vi "Exercise1_Week2.vi"() -> ()   [LabVIEW 2015]
panel:
  out "Output Fibonacci":dbl
  in  "Input Fibonacci":dbl
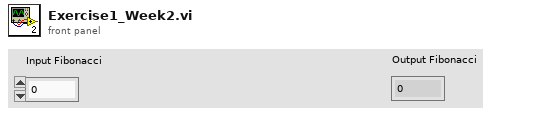
[diagram p1: front panel]
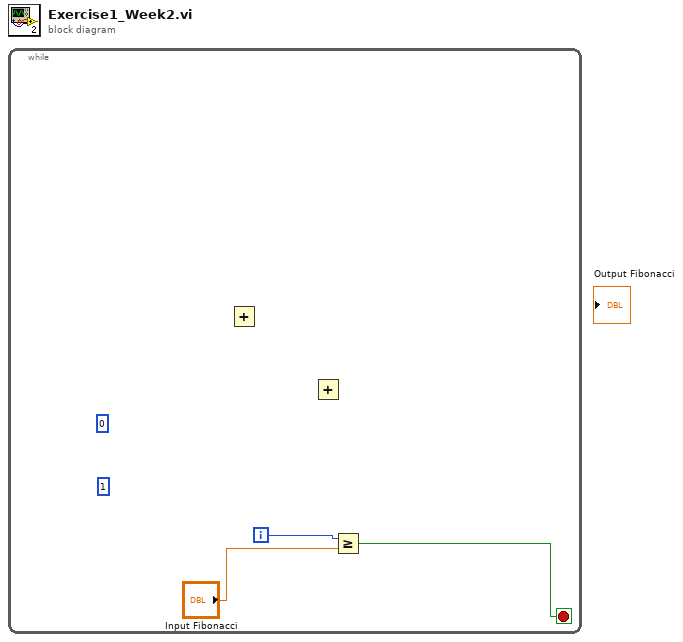
[diagram p0: block diagram]
diagram:
  n1 = while {
    i -> [w2]
    stop <- w3 stop-if-true
    (unwired) 1
    (unwired) 0
    n2 = Add() -> ()  [unwired: 2 in, 1 out]
    n3 = Add() -> ()  [unwired: 2 in, 1 out]
    n4 = Greater Or Equal?(x=w2, y="Input Fibonacci") -> (x >= y?=w3:bool)
  }
